vi "Read Attributes.vi"(11 "Device State Information Msg":refnum<class "Device State Information Msg.lvclass">) -> (2 "Payload":cluster{"Device State Information":T1}={"Device State Information"={"Device State"=enum."DevIDs in Config", "data"=variant}})   [LabVIEW 2018, in "EMS Generic Actor.lvlib" / "Device State Information Msg.lvclass"]
uses:
  Device State Information Msg.lvclass
  EMS Generic/Controls/Device Information Cluster.ctl
  EMS Generic/Controls/Device State.ctl
  Device State Information Msg.lvclass/Device State Information Msg.ctl
  EMS Generic/EMS Generic.lvclass
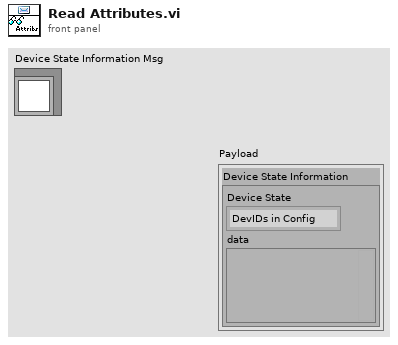
[diagram p1: front panel]
types:
  T1 = typedef "EMS Generic Actor.lvlib/EMS Generic.lvclass/Device Information Cluster.ctl" = cluster{"Device State":T2, "data":variant}
  T2 = typedef "EMS Generic Actor.lvlib/EMS Generic.lvclass/Device State.ctl" = enum16{"Invalid", "Clear", "DevIDs in Config", "DevIDs on uGrid", "DevIDs not on uGrid", "Update IED_Status", "Update DER_Status", "Update DER_Measurement", "Update SmartRelay_Measurement"}
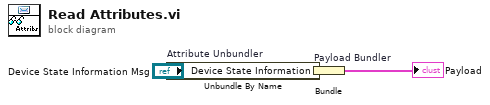
[diagram p0: block diagram]
diagram:
  n1 = Unbundle By Name "Attribute Unbundler"("Device State Information Msg") -> ("Device State Information"=w1:T1)
  n2 = Bundle "Payload Bundler"("Device State Information"=w1) -> (→"Payload":cluster{"Device State Information":T1})  [unwired: 1 in]
